vi "main2 ref.vi"() -> ()   [LabVIEW 2016]
panel:
  in  "VI Refnum":refnum<vi>
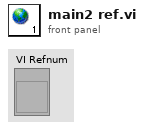
[diagram p1: front panel]
diagram:
